vi "关闭.vi"(8 "error in (no error)":errorcluster caption="错误输入（无错误）", 11 "VISA 输入":refnum<class "VISA.lvclass">) -> (0 "error out":errorcluster caption="错误输出")   [LabVIEW 2016, in "VISA.lvclass"]
uses:
  VISA.lvclass
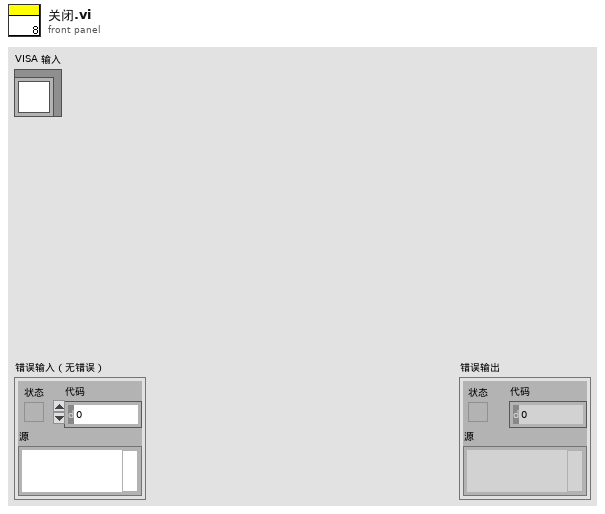
[diagram p1: front panel]
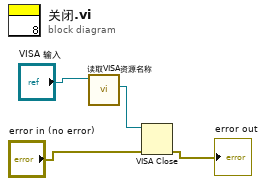
[diagram p0: block diagram]
diagram:
  n1 = call-dynamic "读取VISA资源名称.vi"("VISA输入"="VISA 输入") -> ("VISA资源名称"=w3:refnum<visa-resource-name>)  [unwired: 8 in, 2 out]
  n2 = VISA Close(VISA resource name=w3, error in (no error)="error in (no error)") -> (error out=→"error out":errorcluster)
